vi "UI Network Stream Endpoints.vi"() -> ()   [LabVIEW 2012]
uses:
  controls/UI Data.ctl
panel:
  in  "NS Error Reader":refnum<k21>
  in  "NS Command Writer":refnum<k21>
  # "The NS Command Writer control was created from the writer endpoint terminal of a Create Network Stream Writer Endpoint function with a data type of UI Data.ctl (typedef)."
  # "The NS Error Reader control was created from the reader endpoint terminal of a Create Network Stream Reader Endpoint function with a data type of UI Data.ctl (typedef)."
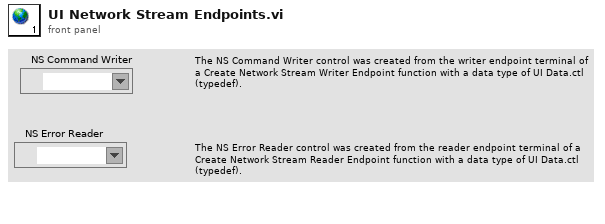
[diagram p1: front panel]
diagram:
